vi "testowy- zabawa kursorami podstawowa.vi"() -> ()   [LabVIEW 2013]
uses:
  <vilib>/measure/NI_MABase.lvlib
  <vilib>/Utility/miscctls.llb/LVCursorListTypeDef.ctl
panel:
  out "Boolean":bool
  out "Position":cluster{"X":dbl, "Y":dbl}
  out "Watch Plots":i32[](array[numeric])
  out "Cursor List":T1
  in  "Slide":i32(slide) scale=0.0..10.0
  in  "stop":bool
  out "Waveform Graph":waveform(dbl)[](graph)
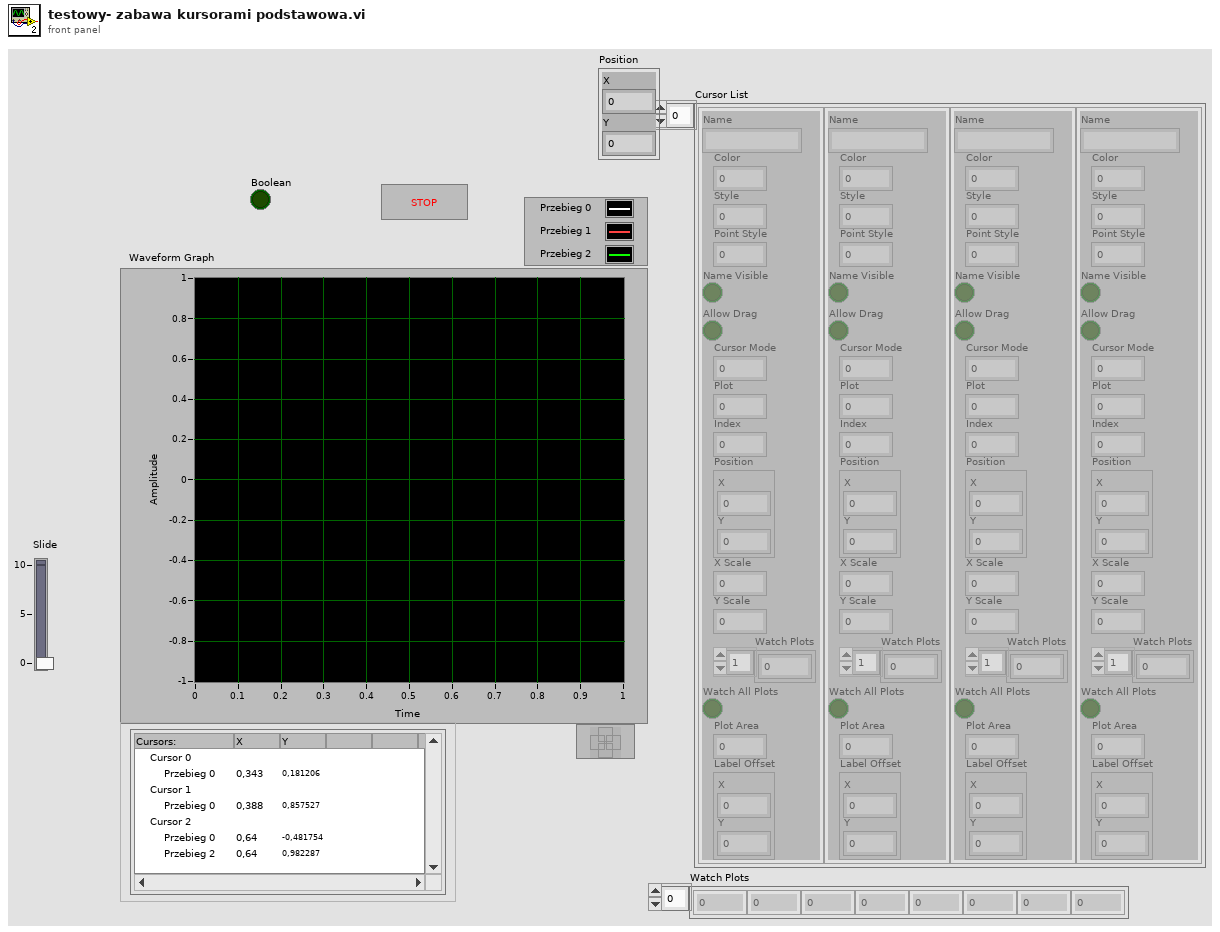
[diagram p1: front panel]
types:
  T1 = typedef "LVCursorListTypeDef.ctl" = cluster{"Name":string, "Color":u32, "Style":u8, "Point Style":u8, "Name Visible":bool, "Allow Drag":bool, "Cursor Mode":u32, "Plot":i32, "Index":i32, "Position":cluster{"X":dbl, "Y":dbl}, "X Scale":u32, "Y Scale":u32, "Watch Plots":i32[], "Watch All Plots":bool, "Plot Area":i32, "Label Offset":cluster{"X":dbl, "Y":dbl}}[]
  T2 = cluster{"Name":string, "Color":u32, "Style":u8, "Point Style":u8, "Name Visible":bool, "Allow Drag":bool, "Cursor Mode":u32, "Plot":i32, "Index":i32, "Position":cluster{"X":dbl, "Y":dbl}, "X Scale":u32, "Y Scale":u32, "Watch Plots":i32[], "Watch All Plots":bool, "Plot Area":i32, "Label Offset":cluster{"X":dbl, "Y":dbl}}
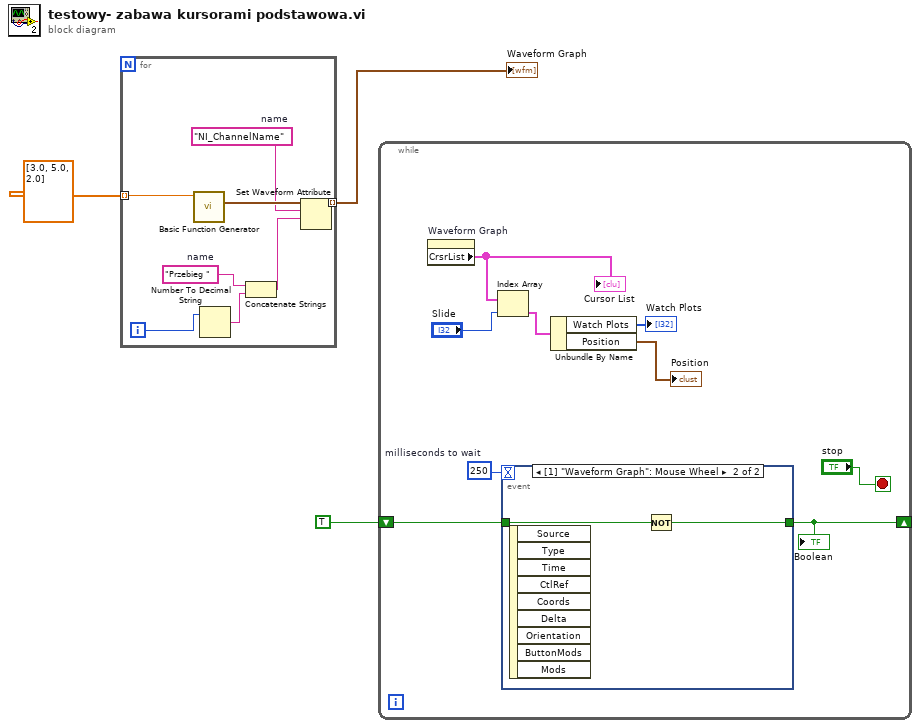
[diagram p0: block diagram]
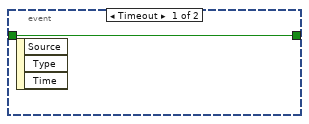
[diagram p2: hidden frame]
diagram:
  n1 = for {
    tunnel: [w10] -> w3 mode=indexing
    tunnel: dbl[] [3.0, 5.0, 2.0] -> [w4] mode=indexing
    i -> [w6]
    w8 = "Przebieg "  # name
    w9 = "NI_ChannelName"  # name
    n2 = call <vilib>:"Basic Function Generator.vi"("frequency"=w4) -> ("signal out"=w11:waveform(dbl))  [unwired: 8 in, 2 out]
    n3 = Number To Decimal String(number=w6) -> (decimal integer string=w5:string)  [unwired: 1 in]
    n4 = Concatenate Strings(w8, w5) -> (w7:string)
    n5 = Set Waveform Attribute(5:w7, 6:w9, 7:w11) -> (3:w10:waveform(dbl))  [unwired: 1 in, 2 out]
  }
  "Waveform Graph" <- w3
  n6 = while {
    shift-right: [w12] -> _
    shift-left: TRUE -> [w13]
    stop <- "stop" stop-if-true
    w14 = u32 250  # milliseconds to wait
    n7 = property on="Waveform Graph" class="WFGraph (strict)"() -> ("CrsrList"=w19:T1)  [unwired: 2 in, 2 out]
    "Cursor List" <- w19
    n8 = Index Array(array=w19, index="Slide") -> (element=w18:T2)
    n9 = event shown="[1] \"Waveform Graph\": Mouse Wheel" {
      selector: _ -> [_ _]
      dyn-events: _ -> [_ _]
      timeout: w14 -> [_ _]
      tunnel: w13 -> [w21 w24]
      tunnel: [w21 w25] -> w12
      event Timeout {
        n10 = event-data() -> ()  [unwired: 1 in, 3 out]
      }
      event "Waveform Graph": Mouse Wheel {
        n11 = event-data() -> ("Delta"=w23:i32, "Orientation"=w22:enum16{"Horizontal", "Vertical"})  [unwired: 1 in, 7 out]
        n12 = Not(x=w24) -> (.not. x?=w25:bool)
      }
    }
    "Boolean" <- w12
    n13 = Unbundle By Name(w18) -> ("Watch Plots"=→"Watch Plots":i32[], "Position"=→"Position":cluster{"X":dbl, "Y":dbl})
  }
